vi "Sim_Position_Tracking.vi"() -> ()   [LabVIEW 2019]
uses:
  Utility_VIs/Position Data.vi
  Sim_Diff_Drive_Globals.vi
panel:
  in  "Zero_XY":bool
  in  "distance(ft)/rotations multiplier":dbl
  out "X and Y pos":cluster{dbl, dbl}(graph)
  out "Pigeon Yaw":cluster{"Yaw":dbl}(graph)
  out "XY Graph":cluster{"array":dbl[], "array":dbl[]}[](graph)
  out "Y position":dbl
  out "X position":dbl
  out "Dist from origin":dbl
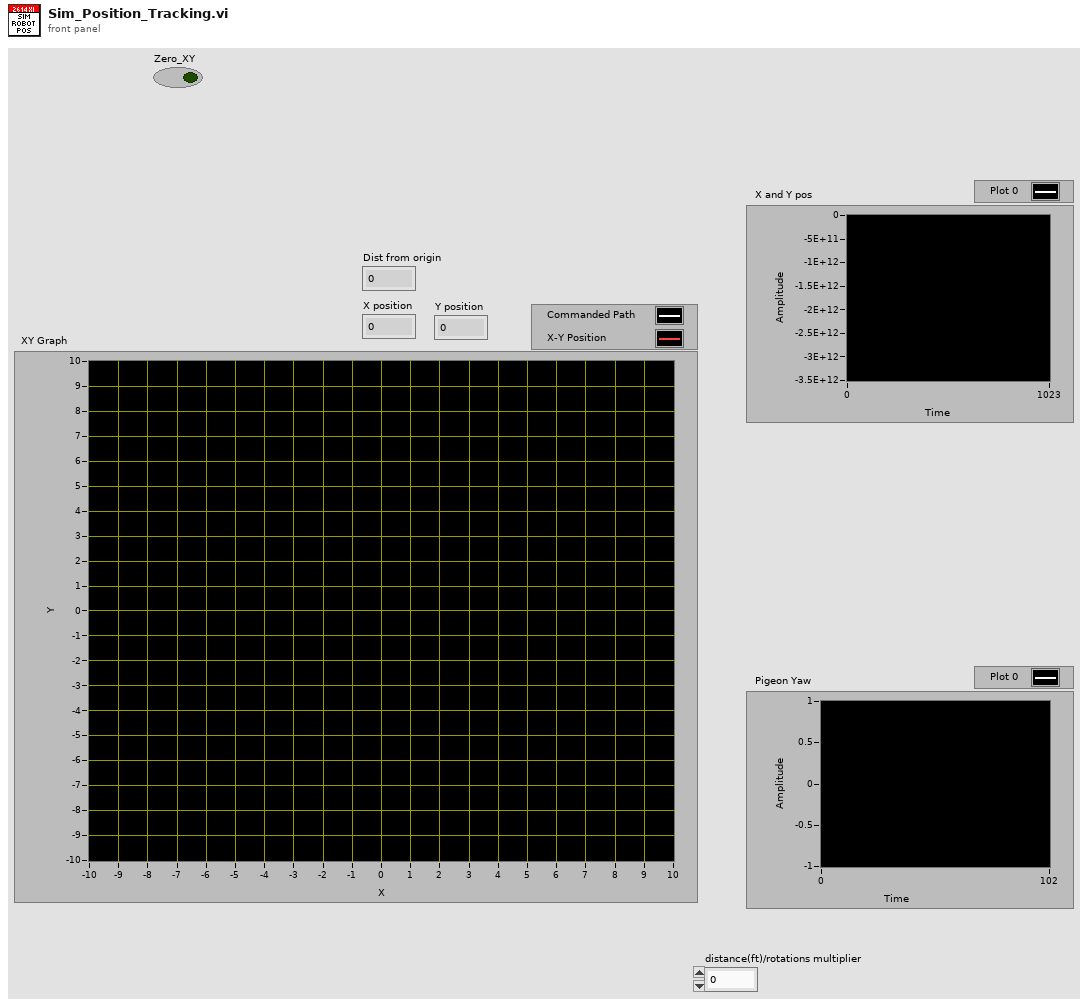
[diagram p1: front panel]
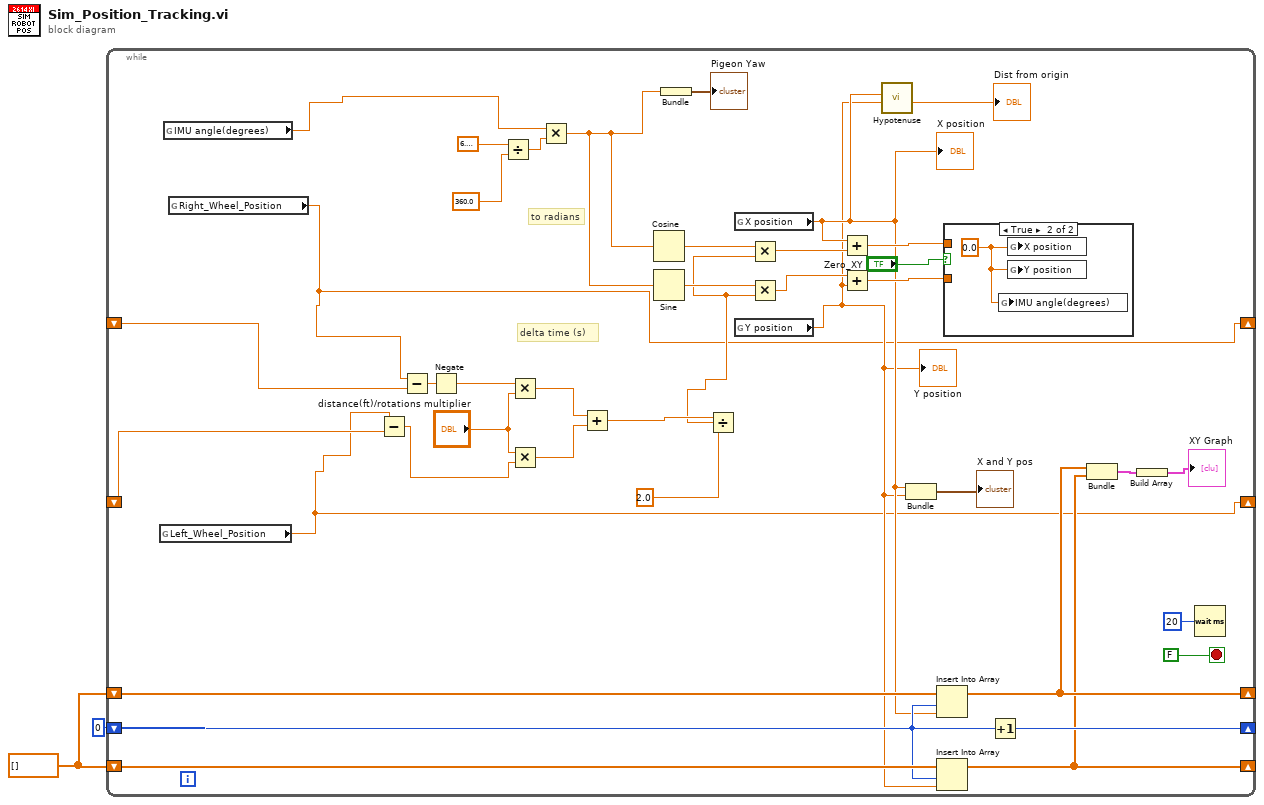
[diagram p0: block diagram]
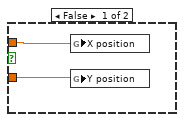
[diagram p2: hidden frame]
diagram:
  w1 = dbl[] [] ("array")
  n1 = while {
    shift-right: [w28] -> _
    shift-left: w1 -> [w32]
    shift-right: [w27] -> _
    shift-left: w1 -> [w31]
    shift-right: [w30] -> _
    shift-left: 0 ("index") -> [w29]
    shift-right: [w5] -> _
    shift-left: _ -> [w8]
    shift-right: [w6] -> _
    shift-left: _ -> [w7]
    stop <- FALSE stop-if-true
    # "to radians"
    # "delta time (s)"
    n2 = global read "Sim_Diff_Drive_Globals.vi" "Left_Wheel_Position"() -> (w6:dbl)
    n3 = global read "Sim_Diff_Drive_Globals.vi" "IMU angle(degrees)"() -> (w4:dbl)
    n4 = global read "Sim_Diff_Drive_Globals.vi" "Right_Wheel_Position"() -> (w5:dbl)
    n5 = Subtract(x=w6, y=w7) -> (x-y=w16:dbl)
    n6 = Subtract(x=w5, y=w8) -> (x-y=w21:dbl)
    n7 = Negate(x=w21) -> (-x=w15:dbl)
    n8 = Divide(x=6.283185307179586, y=360.0) -> (x/y=w22:dbl)
    n9 = Multiply(x=w15, y="distance(ft)/rotations multiplier") -> (x*y=w18:dbl)
    n10 = Multiply(x="distance(ft)/rotations multiplier", y=w16) -> (x*y=w17:dbl)
    n11 = Multiply(x=w4, y=w22) -> (x*y=w14:dbl)
    n12 = Add(x=w18, y=w17) -> (x+y=w20:dbl)
    n13 = Cosine(x=w14) -> (cos(x)=w40:dbl)
    n14 = Sine(x=w14) -> (sin(x)=w38:dbl)
    n15 = Bundle(w14) -> (→"Pigeon Yaw":cluster{dbl})  [unwired: 1 in]
    n16 = Divide(x=w20, y=2.0) -> (x/y=w10:dbl)
    n17 = global read "Position Data.vi" "X position"() -> (w13:dbl)
    "X position" <- w13
    n18 = global read "Position Data.vi" "Y position"() -> (w12:dbl)
    "Y position" <- w12
    n19 = Multiply(x=w40, y=w10) -> (x*y=w39:dbl)
    n20 = Multiply(x=w38, y=w10) -> (x*y=w37:dbl)
    n21 = Add(x=w13, y=w39) -> (x+y=w35:dbl)
    n22 = Add(x=w37, y=w12) -> (x+y=w34:dbl)
    n23 = call "Hypotenuse.vi"("b"=w12, "a"=w13) -> ("c"=→"Dist from origin":dbl)  [unwired: 9 in]
    n24 = Bundle("X position"=w13, "Y position"=w12) -> (→"X and Y pos":cluster{"X position":dbl, "Y position":dbl})  [unwired: 1 in]
    n25 = Insert Into Array(array=w32, index=w29, new element=w13) -> (w28:dbl[])
    n26 = Insert Into Array(array=w31, index=w29, new element=w12) -> (w27:dbl[])
    n27 = case shown="True" "Zero_XY" {
      tunnel: w35 -> [w44 _]
      tunnel: w34 -> [w43 _]
      frame False {
        n28 = global write "Position Data.vi" "X position"(w44) -> ()
        n29 = global write "Position Data.vi" "Y position"(w43) -> ()
      }
      frame True {
        w45 = 0.0 ("X position")
        n30 = global write "Sim_Diff_Drive_Globals.vi" "IMU angle(degrees)"(w45) -> ()
        n31 = global write "Position Data.vi" "X position"(w45) -> ()
        n32 = global write "Position Data.vi" "Y position"(w45) -> ()
      }
    }
    n33 = Increment(x=w29) -> (x+1=w30:i32)
    n34 = Bundle("array"=w28, "array"=w27) -> (w26:cluster{"array":dbl[], "array":dbl[]})  [unwired: 1 in]
    n35 = Build Array(w26) -> (→"XY Graph":cluster{"array":dbl[], "array":dbl[]}[])
    n36 = Wait (ms)(milliseconds to wait=u32 20) -> ()  [unwired: 1 out]
  }
